vi "SendJson.vi"(8 "error in (no error)":errorcluster, 9 "timeout":i32=-1, 10 "String Data":string, 11 "Communicator in":refnum<class "Communicator.lvclass">) -> (0 "error out":errorcluster, 3 "Communicator out":refnum<class "Communicator.lvclass">)   [LabVIEW 2023, in "Communicator.lvclass"]
uses:
  Communicator.lvclass
  Communicator.lvclass/Communicator.ctl
  <vilib>/MediaMongrels Ltd/WebSockets/WebSockets/WebSocket Client/WebSocket Client.lvclass
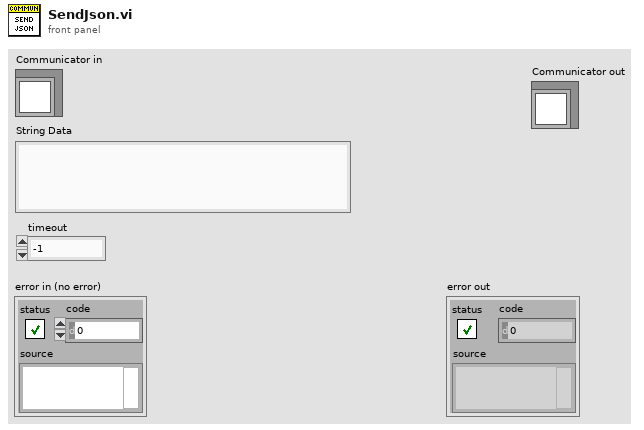
[diagram p1: front panel]
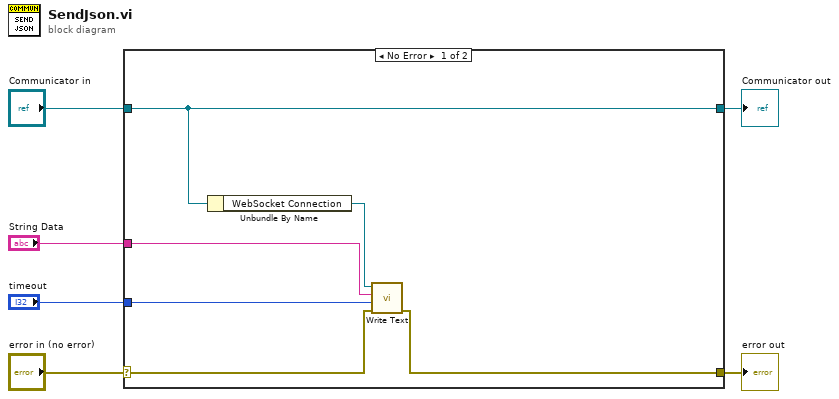
[diagram p0: block diagram]
diagram:
  n1 = case shown="No Error" "error in (no error)" {
    selector: "error in (no error)" -> [w11 w14]
    tunnel: [w10 w14] -> w5
    tunnel: [w8 w13] -> w3
    tunnel: "Communicator in" -> [w8 w13]
    tunnel: "timeout" -> [w12 _]
    tunnel: "String Data" -> [w9 _]
    frame No Error {
      n2 = Unbundle By Name(w8) -> ("WebSocket Connection"=w7:refnum<class "WebSocket Client.lvclass">)
      n3 = call-dynamic "Write Text.vi"("error in (no error)"=w11, "timeout ms (5000)"=w12, "String Data"=w9, "WebSocket in"=w7) -> ("error out"=w10:errorcluster)  [unwired: 6 in, 1 out]
    }
    frame Error {
    }
  }
  "error out" <- w5
  "Communicator out" <- w3
